vi "Authorization Decode XML.vi"(8 "error in (no error)":errorcluster, 10 "RootPathName (C:\\)":string="C:\\", 11 "Encoded XML String":string) -> (0 "error out":errorcluster, 2 "Valid":bool, 3 "Decoded XML String":string)   [LabVIEW 2011]
uses:
  <vilib>/xml/Load XML String.vi
  <vilib>/xml/Close Reference(Node).vi
  <vilib>/xml/NI_XML.lvlib
  LabVIEW 2011/resource/objmgr/DOMUserDefRef.rc
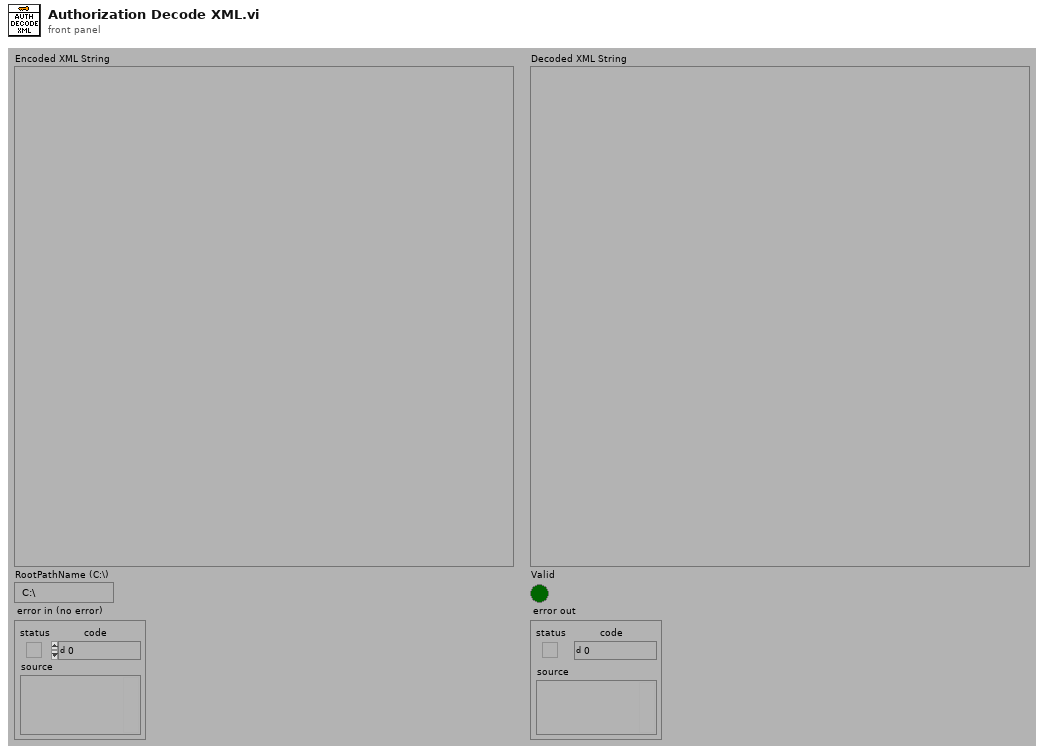
[diagram p1: front panel]
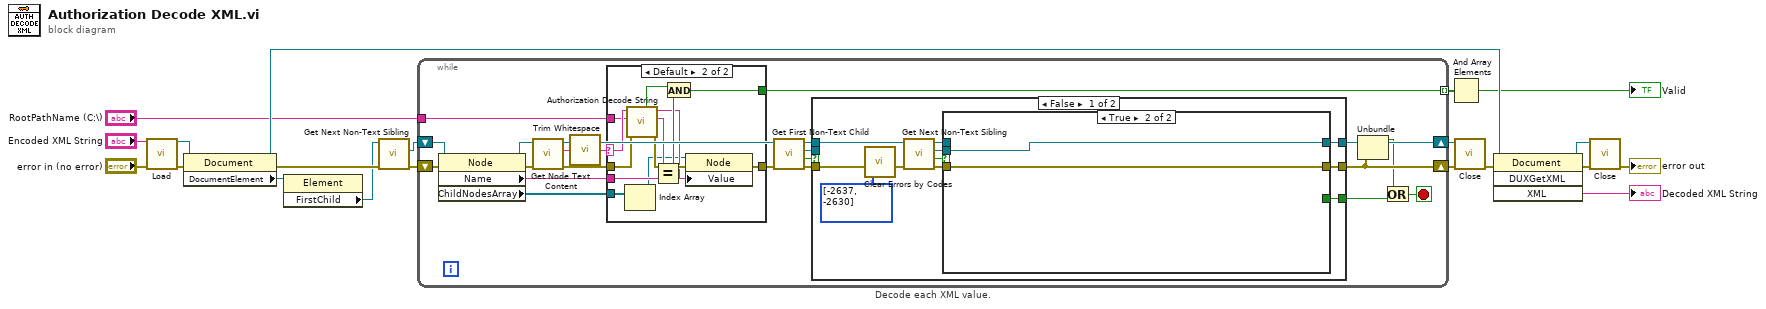
[diagram p0: block diagram]
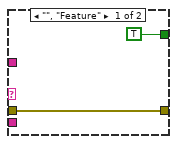
[diagram p2: hidden frame]
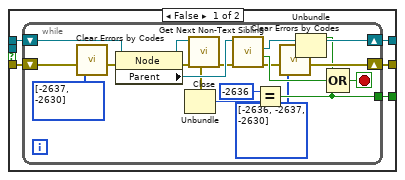
[diagram p3: hidden frame]
diagram:
  n1 = call-poly <vilib>:"Load.vi"("XML string"="Encoded XML String", "error in (no error)"="error in (no error)") -> ("DOM document out"=w20:refnum<k20>, "error out"=w19:errorcluster)  [unwired: 11 in, 1 out]
  n2 = property on="Property Node" class="Document"(reference=w20, error in=w19) -> (reference out=w11:refnum<k20>, error out=w17:errorcluster, "DocumentElement"=w18:refnum<k20>)
  n3 = property on="Property Node" class="Element"(reference=w18) -> ("FirstChild"=w16:refnum<k20>)  [unwired: 1 in, 2 out]
  n4 = call <vilib>:"Get Next Non-Text Sibling.vi"("error in (no error)"=w17, "node in"=w16) -> ("error out"=w15:errorcluster, "sibling node"=w14:refnum<k20>)  [unwired: 6 in, 2 out]
  n5 = while "Decode each XML value." {
    shift-right: [w26] -> w13
    shift-left: w15 -> [w36]
    shift-right: [w42] -> w12
    shift-left: w14 -> [w33]
    tunnel: [w27] -> w3 mode=indexing
    tunnel: "RootPathName (C:\\)" -> [w21]
    stop <- w28 stop-if-true
    n6 = property class="Node"(reference=w33, error in=w36) -> (reference out=w32:refnum<k20>, error out=w35:errorcluster, "Name"=w41:string, "ChildNodesArray"=w22:refnum<k20>[])
    n7 = call <vilib>:"Get Node Text Content.vi"("error in (no error)"=w35, "node in"=w32) -> ("error out"=w34:errorcluster, "node text"=w24:string, "node out"=w30:refnum<k20>)  [unwired: 7 in]
    n8 = call <vilib>:"Trim Whitespace.vi"("string"=w24) -> ("trimmed string"=w23:string)  [unwired: 1 in]
    n9 = case shown="Default" w23 {
      selector: w23 -> [_ w48]
      tunnel: w41 -> [_ w55]
      tunnel: w34 -> [w44 w51]
      tunnel: [w44 w50] -> w29
      tunnel: [TRUE w49] -> w27
      tunnel: w22 -> [_ w47]
      tunnel: w21 -> [_ w45]
      frame "", "Feature" {
      }
      frame Default {
        n10 = Index Array(array=w47) -> (element=w46:refnum<k20>)  [unwired: 1 in]
        n11 = call "Authorization Decode String.vi"("error in (no error)"=w51, "RootPathName (C:\\)"=w45, "Encoded String"=w48) -> ("error out"=w53:errorcluster, "Property Name"=w54:string, "Decoded String"=w52:string, "Valid?"=w56:bool)  [unwired: 3 in, 2 out]
        n12 = Equal?(x=w54, y=w55) -> (x = y?=w57:bool)
        n13 = And(x=w56, y=w57) -> (x .and. y?=w49:bool)
        n14 = property class="Node"(reference=w46, error in=w53, "Value"=w52) -> (error out=w50:errorcluster)  [unwired: 1 out]
      }
    }
    n15 = call <vilib>:"Get First Non-Text Child.vi"("error in (no error)"=w29, "node in"=w30) -> ("error out"=w39:errorcluster, "found child node?"=w40:bool, "child node"=w38:refnum<k20>, "node out"=w37:refnum<k20>)  [unwired: 6 in]
    n16 = case shown="False" w40 {
      tunnel: w39 -> [w60 w94]
      tunnel: w38 -> [_ w95]
      tunnel: w37 -> [w68 _]
      tunnel: [w63 w95] -> w42
      tunnel: [w64 w94] -> w26
      tunnel: [w61 _] -> w31
      frame False {
        n17 = call "Clear Errors by Codes.vi"("Error Codes\nto Clear (Empty)"=i32[] [-2637, -2630], "error in (no error)"=w60) -> ("error out"=w59:errorcluster)  [unwired: 5 in]
        n18 = call <vilib>:"Get Next Non-Text Sibling.vi"("error in (no error)"=w59, "node in"=w68) -> ("error out"=w67:errorcluster, "found sibling node?"=w66:bool, "sibling node"=w65:refnum<k20>, "node out"=w62:refnum<k20>)  [unwired: 6 in]
        n19 = case shown="True" w66 {
          tunnel: w67 -> [w69 w93]
          tunnel: w65 -> [_ w92]
          tunnel: [w71 w93] -> w64
          tunnel: [w72 w92] -> w63
          tunnel: w62 -> [w73 _]
          tunnel: [w70 _] -> w61
          frame False {
            n20 = while {
              shift-right: [w88] -> w72
              shift-left: w73 -> [w91]
              shift-right: [w75] -> w71
              shift-left: w69 -> [w82]
              tunnel: [w80] -> w70
              stop <- w86 stop-if-true
              n21 = call "Clear Errors by Codes.vi"("Error Codes\nto Clear (Empty)"=i32[] [-2637, -2630], "error in (no error)"=w82) -> ("error out"=w81:errorcluster)  [unwired: 5 in]
              n22 = property class="Node"(reference=w91, error in=w81) -> (reference out=w90:refnum<k20>, error out=w76:errorcluster, "Parent"=w89:refnum<k20>)
              n23 = Unbundle(w76) -> ("code"=w84:i32)  [unwired: 2 out]
              n24 = call-poly <vilib>:"Close.vi"("error in (no error)"=w76, "node"=w90) -> ("error out"=w77:errorcluster)  [unwired: 7 in]
              n25 = call <vilib>:"Get Next Non-Text Sibling.vi"("error in (no error)"=w77, "node in"=w89) -> ("error out"=w78:errorcluster, "found sibling node?"=w87:bool, "sibling node"=w88:refnum<k20>)  [unwired: 6 in, 1 out]
              n26 = Equal?(x=-2636, y=w84) -> (x = y?=w80:bool)
              n27 = call "Clear Errors by Codes.vi"("Error Codes\nto Clear (Empty)"=i32[] [-2636, -2637, -2630], "error in (no error)"=w78) -> ("error out"=w75:errorcluster)  [unwired: 5 in]
              n28 = Unbundle(w75) -> ("status"=w74:bool)  [unwired: 2 out]
              n29 = Compound Arithmetic op=OR(w74, w87, w80) -> (w86:bool)
            }
          }
          frame True {
          }
        }
      }
      frame True {
      }
    }
    n30 = Unbundle(w26) -> ("status"=w25:bool)  [unwired: 2 out]
    n31 = Or(x=w25, y=w31) -> (x .or. y?=w28:bool)
  }
  n32 = And Array Elements(Boolean array=w3) -> (logical AND=→"Valid":bool)
  n33 = call-poly <vilib>:"Close.vi"("error in (no error)"=w13, "node"=w12) -> ("error out"=w10:errorcluster)  [unwired: 7 in]
  n34 = invoke class="Document" method="DUXGetXML"(reference=w11, error in=w10) -> (reference out=w8:refnum<k20>, error out=w9:errorcluster, "XML"=→"Decoded XML String":string)  [unwired: 2 in, 1 out]
  n35 = call-poly <vilib>:"Close.vi"("error in (no error)"=w9, "node"=w8) -> ("error out"=→"error out":errorcluster)  [unwired: 7 in]
